vi "AlliGator Compute Parameters SDV.vi"(0 "Parameters in":dbl[](array[numeric]), 2 "Reference Phasor 1":T1, 3 "Reference Phasor 2":T1, 5 "Phasor":cluster{"g":dbl, "s":dbl}, 7 "Phasor Frequency":dbl[unit], 9 "Raw Phasor SDV":T1, 11 "error in (no error)":errorcluster, 12 "Calibration Phasor":T2, 13 "Reference Lifetime 1":dbl[unit], 14 "Reference Lifetime 2":dbl[unit]) -> (4 "Parameters out":dbl[](array[numeric]), 15 "error out":errorcluster)   [LabVIEW 2021, in "AlliGator Phasor Graph.lvlib"]
doc: "Computes average and SDV of phasor-related quantities."
uses:
  AlliGator Phasor Graph.lvlib
  Phasor/Phasor (g, s).ctl
  Phasor/Calibration Phasor (m, phi).ctl
  Phasor/Phasor (m, phi).ctl
  df9727a4-955e-4024-8cdf-5e236669f78b.vi
  df9727a4-955e-4024-8cdf-5e236669f78b.vi/8a80743f-1319-44c8-96b0-3ef8fc688731.vi
  df9727a4-955e-4024-8cdf-5e236669f78b.vi/931f4f8f-d8c6-4056-833f-5c8fe97b24b9.vi
  Phasor/Phasor.lvlib
panel:
  # "see the AlliGator License on the block diagram (Ctrl+E or Window:Show Block Diagram)"
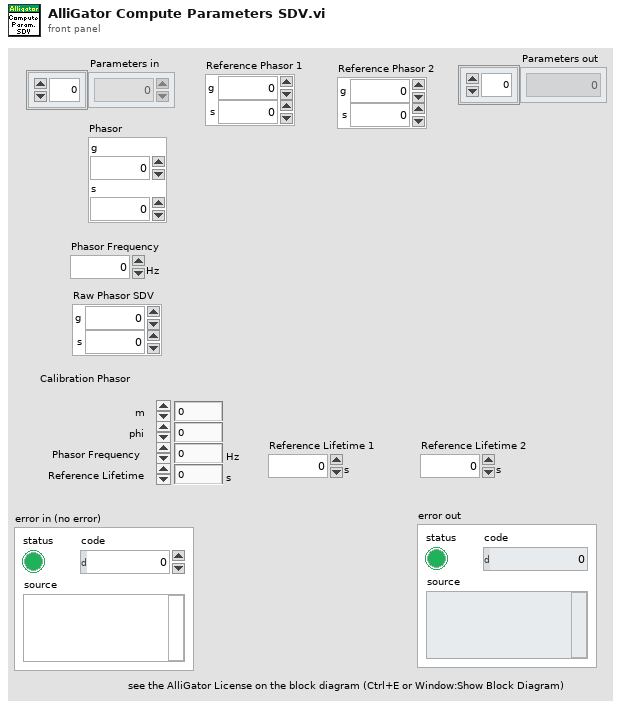
[diagram p1: front panel]
types:
  T1 = typedef "Phasor.lvlib/Phasor (g, s).ctl" = cluster{"g":dbl, "s":dbl}
  T2 = typedef "Phasor.lvlib/Calibration Phasor (m, phi).ctl" = cluster{"m":dbl, "phi":dbl, "Phasor Frequency":dbl[unit], "Reference Lifetime":dbl[unit]}
  T3 = typedef "Phasor.lvlib/Phasor (m, phi).ctl" = cluster{"m":dbl, "phi":dbl}
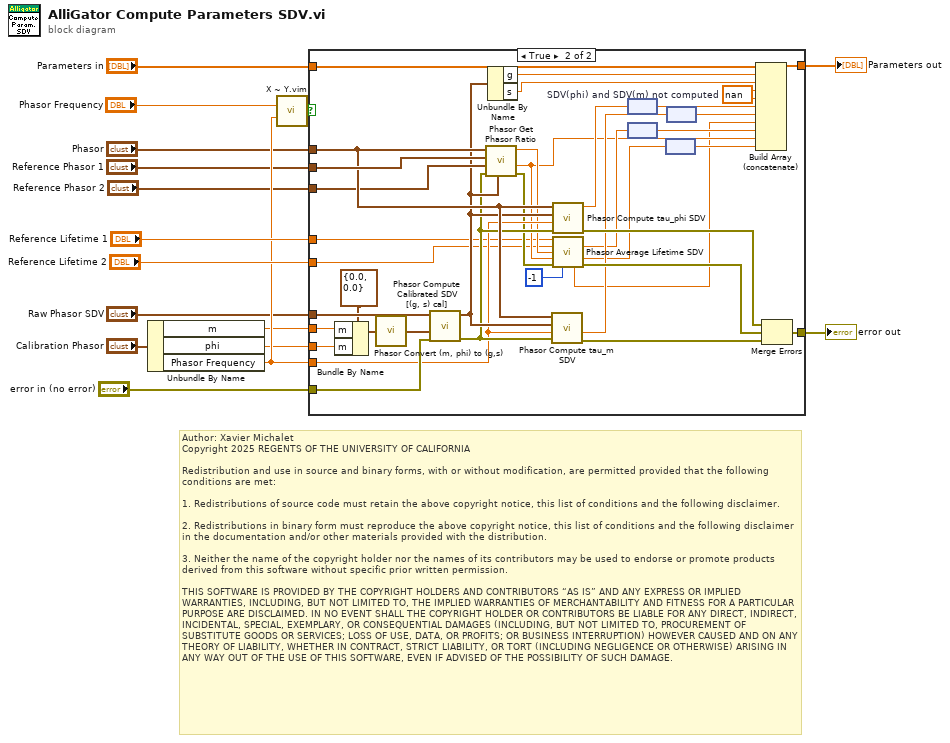
[diagram p0: block diagram]
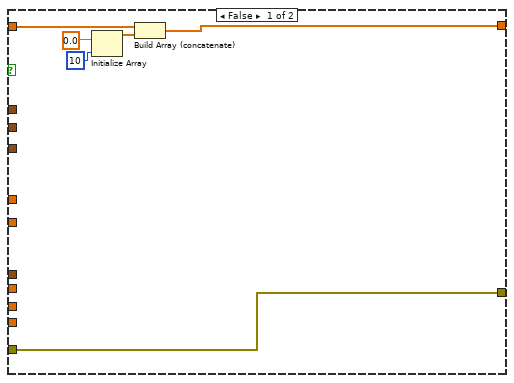
[diagram p2: hidden frame]
diagram:
  # "Author: Xavier Michalet\nCopyright 2025 REGENTS OF THE UNIVERSITY OF CALIFORNIA\n\nRedistribution and use in source and binary forms, with or without modification, are permitted provided that the following conditions are met:\n\n1. Redistributions of source code must retain the above copyright notice, this list of conditions and the following disclaimer.\n\n2. Redistributions in binary form must reproduce the above copyright notice, this list of conditions and the following disclaimer in the documentation and/or other materials provided with the distribution.\n\n3. Neither the name of the copyright holder nor the names of its contributors may be used to endorse or promote products derived from this software without specific prior written permission.\n\nTHIS SOFTWARE IS PROVIDED BY THE COPYRIGHT HOLDERS AND CONTRIBUTORS “AS IS” AND ANY EXPRESS OR IMPLIED WARRANTIES, INCLUDING, BUT NOT LIMITED TO, THE IMPLIED WARRANTIES OF MERCHANTABILITY AND FITNESS FOR A PARTICULAR PURPOSE ARE DISCLAIMED. IN NO EVENT SHALL THE COPYRIGHT HOLDER OR CONTRIBUTORS BE LIABLE FOR ANY DIRECT, INDIRECT, INCIDENTAL, SPECIAL, EXEMPLARY, OR CONSEQUENTIAL DAMAGES (INCLUDING, BUT NOT LIMITED TO, PROCUREMENT OF SUBSTITUTE GOODS OR SERVICES; LOSS OF USE, DATA, OR PROFITS; OR BUSINESS INTERRUPTION) HOWEVER CAUSED AND ON ANY THEORY OF LIABILITY, WHETHER IN CONTRACT, STRICT LIABILITY, OR TORT (INCLUDING NEGLIGENCE OR OTHERWISE) ARISING IN ANY WAY OUT OF THE USE OF THIS SOFTWARE, EVEN IF ADVISED OF THE POSSIBILITY OF SUCH DAMAGE."
  n1 = Unbundle By Name("Calibration Phasor") -> ("m"=w5:dbl, "phi"=w6:dbl, "Phasor Frequency"=w14:dbl[unit])
  n2 = call "X ~ Y.vim"("X"="Phasor Frequency", "Y"=w14) -> ("X ~= Y?"=w8:bool)  [unwired: 13 in]
  n3 = case shown="True" w8 {
    tunnel: "Parameters in" -> [w19 w59]
    tunnel: [w18 w58] -> w2
    tunnel: "Raw Phasor SDV" -> [_ w57]
    tunnel: w5 -> [_ w55]
    tunnel: w6 -> [_ w54]
    tunnel: "error in (no error)" -> [w17 w34]
    tunnel: [w17 w27] -> w10
    tunnel: "Phasor" -> [_ w37]
    tunnel: "Reference Phasor 1" -> [_ w38]
    tunnel: "Reference Phasor 2" -> [_ w36]
    tunnel: w14 -> [_ w32]
    tunnel: "Reference Lifetime 1" -> [_ w26]
    tunnel: "Reference Lifetime 2" -> [_ w25]
    frame False {
      n4 = Initialize Array(0.0 ("Numeric Control"), 10 ("dimension size")) -> (w22:dbl[])
      n5 = Build Array (concatenate)(w19, w22) -> (w18:dbl[])
    }
    frame True {
      w50 = nan  # SDV(phi) and SDV(m) not computed
      n6 = Bundle By Name(cluster=T3 {"m"=0.0, "phi"=0.0} ("Phasor (m, phi)"), "m"=w55, "m"=w54) -> (w52:T3)
      n7 = call "Phasor Convert (m, phi) to (g,s).vi"("Phasor (m, phi)"=w52) -> ("Phasor (g, s)"=w56:T1)  [unwired: 8 in]
      n8 = call "Phasor Compute Calibrated SDV [(g, s) cal].vi"("Error In"=w34, "Phasor Calibration (g,s)"=w56, "Raw Phasor SDV (g, s)"=w57) -> ("Error Out"=w33:errorcluster, "Calibrated Phasor SDV (g, s)"=w35:T1)  [unwired: 7 in]
      n9 = call "Phasor Get Phasor Ratio.vi"("Phasor SDV"=w35, "Error In"=w33, "Reference Phasor 2"=w36, "Reference Phasor 1"=w38, "Phasor"=w37) -> ("Error Out"=w31:errorcluster, "Phasor Ratio SDV"=w29:dbl, "Phasor Ratio (f1)"=w30:dbl)  [unwired: 4 in]
      n10 = Unbundle By Name(w35) -> ("g"=w51:dbl, "s"=w24:dbl)
      n11 = call "Phasor Compute tau_m SDV.vi"("Error In"=w33, "Phasor Frequency"=w32, "Phasor SDV (g, s)"=w35, "Phasor (g, s)"=w37) -> ("Error Out"=w47:errorcluster, "tau_m SDV"=w44:dbl[unit])  [unwired: 5 in, 1 out]
      n12 = call "Phasor Compute tau_phi SDV.vi"("Error In"=w33, "Phasor Frequency"=w32, "Phasor SDV (g, s)"=w35, "Phasor (g, s)"=w37) -> ("Error Out"=w49:errorcluster, "tau_phi SDV"=w46:dbl[unit])  [unwired: 6 in]
      n13 = call "Phasor Average Lifetime SDV.vi"("tau 1"=w26, "tau 2"=w25, "r"=w30, "SDV r"=w29, "Error In"=w31, "seed"=-1) -> ("SDV <tau>_a"=w42:dbl[unit], "SDV <tau>_i"=w41:dbl[unit], "SDV a"=w28:dbl, "Error Out"=w48:errorcluster)  [unwired: 4 in, 2 out]
      n14 = node(w46) -> (w45:dbl)
      n15 = node(w42) -> (w40:dbl)
      n16 = node(w41) -> (w39:dbl)
      n17 = node(w44) -> (w43:dbl)
      n18 = Build Array (concatenate)(w59, w51, w24, w50, w50, w45, w43, w28, w40, w29, w39) -> (w58:dbl[])
      n19 = Merge Errors(w49, w48, w47) -> (w27:errorcluster)
    }
  }
  "error out" <- w10
  "Parameters out" <- w2
